vi "Display Measurements.vi"(8 "error in (no error)":errorcluster, 11 "Controller in":refnum<class "Controller.lvclass">) -> (0 "error out":errorcluster, 3 "Controller out":refnum<class "Controller.lvclass">)   [LabVIEW 2016, in "Controller Actor.lvlib" / "Controller.lvclass"]
uses:
  <userlib>/Common Components/Controller/Controller.lvclass
  <userlib>/Common Components/Controller UI/Messages/List of Measurements Message/List of Measurements Message.lvclass
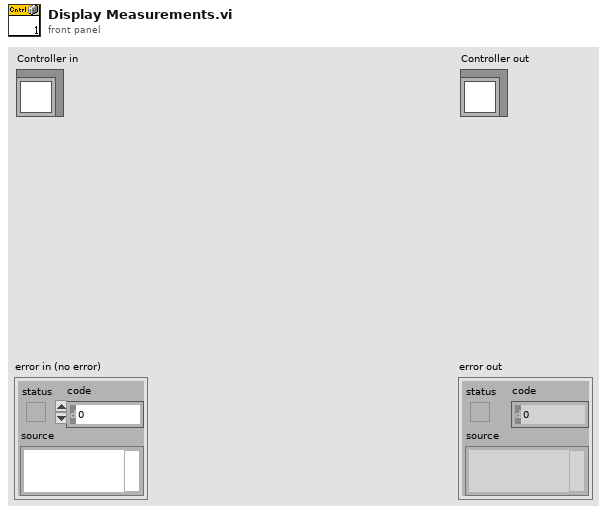
[diagram p1: front panel]
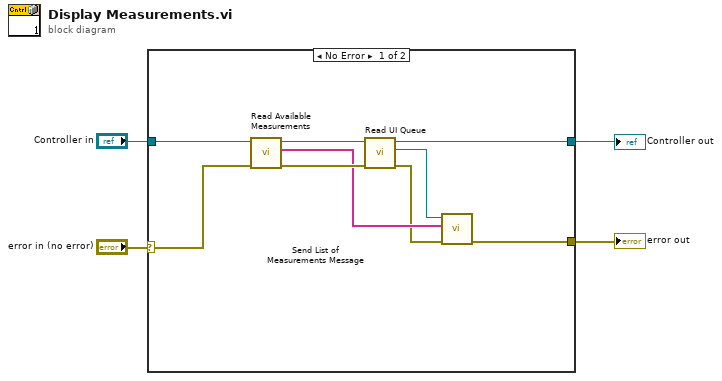
[diagram p0: block diagram]
diagram:
  n1 = case shown="No Error" "error in (no error)" {
    selector: "error in (no error)" -> [w12 w15]
    tunnel: [w5 w15] -> w3
    tunnel: [w9 w14] -> w1
    tunnel: "Controller in" -> [w13 w14]
    frame No Error {
      n2 = call <userlib>:"Read Available Measurements.vi"("error in (no error)"=w12, "Controller in"=w13) -> ("error out"=w8:errorcluster, "Available Measurements"=w7:string[], "Controller out"=w10:refnum<class "Controller.lvclass">)  [unwired: 7 in]
      n3 = call <userlib>:"Read UI Queue.vi"("error in (no error)"=w8, "UI Controller in"=w10) -> ("error out"=w6:errorcluster, "UI Queue"=w11:refnum<class "Message Enqueuer.lvclass">, "UI Controller out"=w9:refnum<class "Controller.lvclass">)  [unwired: 7 in]
      n4 = call <userlib>:"Send List of Measurements Message.vi"("error in (no error)"=w6, "List of Measurement Names"=w7, "Message Enqueuer in"=w11) -> ("error out"=w5:errorcluster)  [unwired: 7 in, 1 out]
    }
    frame Error {
    }
  }
  "error out" <- w3
  "Controller out" <- w1
